vi "Init(SGL).vi"(8 "错误输入":errorcluster, 11 "TagList":T1[](array[typedef])) -> (0 "错误输出":errorcluster)   [LabVIEW 2013, in "Tag Data by Variant.lvlib"]
uses:
  Tag Data by Variant.lvlib
  Custom def/Tag SGL.ctl
  Custom def/mode.ctl
  Core/TagVar Data(SGL).vi
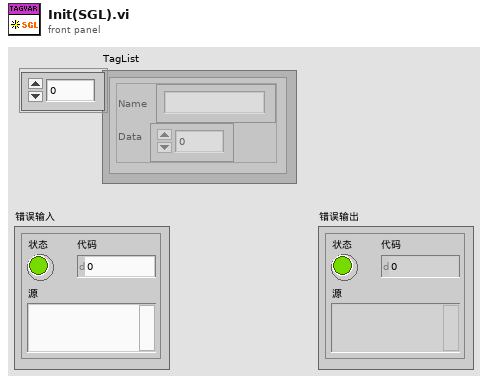
[diagram p1: front panel]
types:
  T1 = typedef "Tag Data by Variant.lvlib/Tag SGL.ctl" = cluster{"Name":string, "Data":sgl}
  T2 = typedef "Tag Data by Variant.lvlib/mode.ctl" = enum16{"初始化", "加入", "删除", "读取", "读取所有", "清除"}
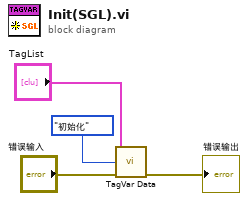
[diagram p0: block diagram]
diagram:
  n1 = call-poly "TagVar Data.vi"("错误输入"="错误输入", "method"=mode."初始化", "TagList"="TagList") -> ("错误输出"=→"错误输出":errorcluster)  [unwired: 6 in, 2 out]
